vi "Parse-element.vi"(8 "error in (no error)":errorcluster, 10 "String in":string, 11 "Element-XML in":refnum<class "EndJob.lvclass">) -> (0 "error out":errorcluster, 1 "Valid element?":bool, 2 "Remaining string":string, 3 "Element-XML out":refnum<class "EndJob.lvclass">)   [LabVIEW 2013, in "HardwareCharacterization.lvlib" / "EndJob.lvclass"]
uses:
  EndJob.lvclass
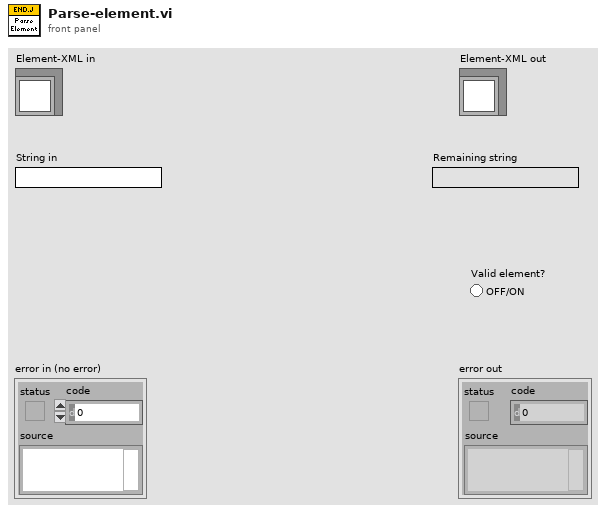
[diagram p1: front panel]
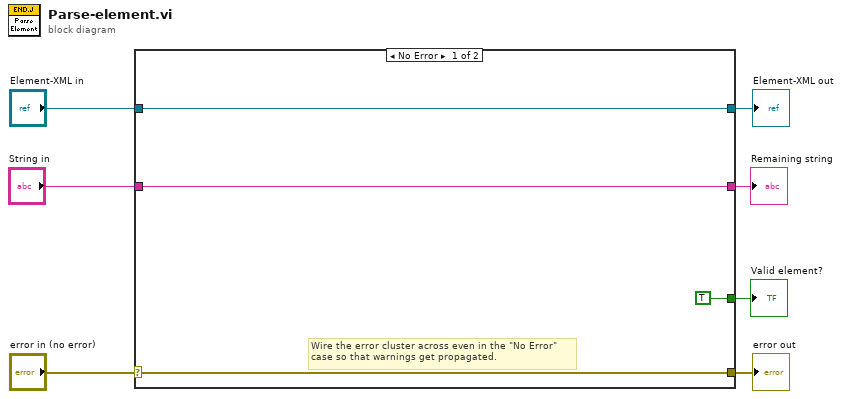
[diagram p0: block diagram]
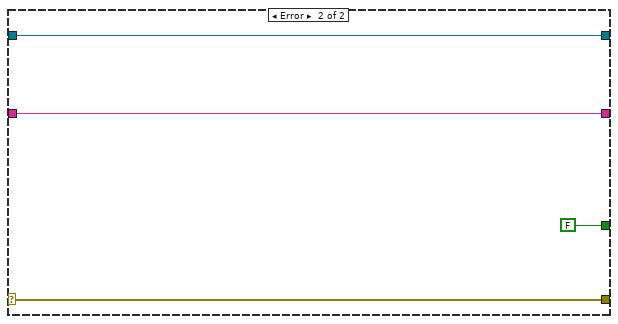
[diagram p2: hidden frame]
diagram:
  n1 = case shown="No Error" "error in (no error)" {
    selector: "error in (no error)" -> [w10 w15]
    tunnel: [w10 w15] -> w6
    tunnel: [w11 w14] -> w4
    tunnel: "Element-XML in" -> [w11 w14]
    tunnel: "String in" -> [w8 w12]
    tunnel: [TRUE FALSE] -> w2
    tunnel: [w8 w12] -> w1
    frame No Error {
      # "Wire the error cluster across even in the \"No Error\"\ncase so that warnings get propagated."
    }
    frame Error {
    }
  }
  "error out" <- w6
  "Element-XML out" <- w4
  "Valid element?" <- w2
  "Remaining string" <- w1
